vi "Sound Alert.vi"   [LabVIEW 2022 SP3]
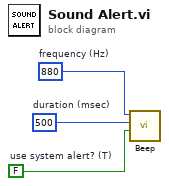
[diagram p0: block diagram]
diagram:
  w3 = FALSE  # use system alert? (T)
  w2 = u32 500  # duration (msec)
  w1 = u32 880  # frequency (Hz)
  n1 = call <vilib>:"Beep.vi"("use system alert? (T)"=w3, "duration (msec)"=w2, "frequency (Hz)"=w1) -> ()  [unwired: 9 in]
